vi "GlobalClicksHeight_flt.vi"() -> ()   [LabVIEW 2019]
panel:
  out "pen pos":cluster{"X":dbl, "Z":dbl, "y scaled":dbl}
  out "Frame Properties":cluster{"FH":dbl, "FW":dbl, "Origin":dbl}
  in  "Safe Tip?":bool
  in  "Starting Height (nm)":dbl
  out "Setpoint (A)":dbl=100.0
  out "Current (pA)":dbl
  in  "Found Surface?":bool
  out "Surface Location (nm)":dbl
  in  "Starting Height?":bool
  in  "Clicks and Height":bool
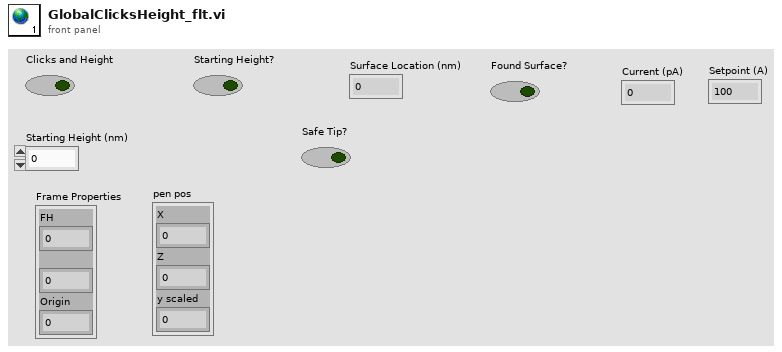
[diagram p1: front panel]
diagram:
